vi "Custom.vi"(8 "error in (no error)":errorcluster, 11 "Transport Parameters in":T1 {"Serial Communication"."Baud Rate" items=["75"=75, "110"=110, "134"=134, "150"=150, "300"=300, "600"=600, "1200"=1200, "1800"=1800, "2400"=2400, "4800"=4800, "7200"=7200, "9600"=9600, "14400"=14400, "19200"=19200, "28800"=28800, "38400"=38400, "56000"=56000, "57600"=57600, "115200"=115200, "128000"=128000, "230400"=230400]}) -> (0 "error out":errorcluster, 3 "Transport Parameters out":T1 {"Serial Communication"."Baud Rate" items=["75"=75, "110"=110, "134"=134, "150"=150, "300"=300, "600"=600, "1200"=1200, "1800"=1800, "2400"=2400, "4800"=4800, "7200"=7200, "9600"=9600, "14400"=14400, "19200"=19200, "28800"=28800, "38400"=38400, "56000"=56000, "57600"=57600, "115200"=115200, "128000"=128000, "230400"=230400]})   [LabVIEW 2020]
uses:
  Controls/ConnectionParameters.ctl
  Controls/SupportedTransports.ctl
panel:
  out "spreadsheet string":string
  out "Message Out":string
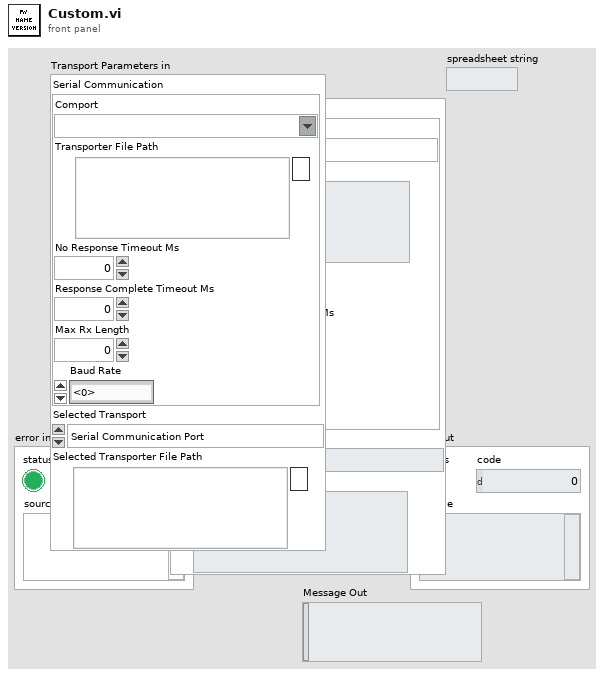
[diagram p1: front panel]
types:
  T1 = typedef "ConnectionParameters.ctl" = cluster{"Serial Communication":cluster{"Comport":refnum<visa-resource-name>, "Transporter File Path":path, "No Response Timeout Ms":u32, "Response Complete Timeout Ms":u32, "Max Rx Length":u32, "Baud Rate":u32}, "Selected Transport":T2, "Selected Transporter File Path":path}
  T2 = typedef "SupportedTransports.ctl" = enum16{"Serial Communication Port"}
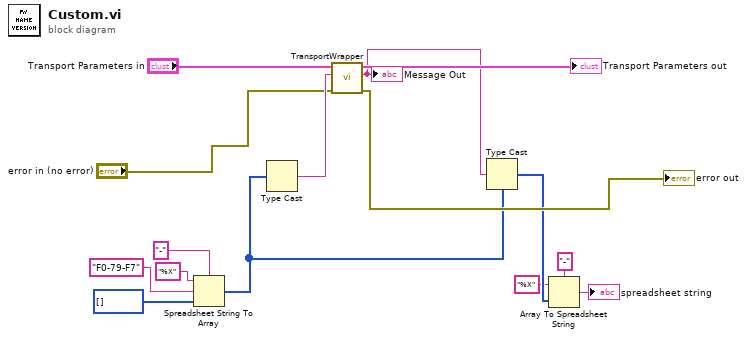
[diagram p0: block diagram]
diagram:
  n1 = Spreadsheet String To Array(delimiter (Tab)="-", format string="%X", spreadsheet string="F0-79-F7" ("Message In"), array type (2D Dbl)=u8[] []) -> (array=w5:u8[])
  n2 = Type Cast(x=w5) -> (*(type *) &x=w15:string)  [unwired: 1 in]
  n3 = call "TransportWrapper.vi"("error in"="error in (no error)", "Message In"=w15, "Transport Parameters In"="Transport Parameters in") -> ("error out"=→"error out":errorcluster, "Message Out"=w6:string, "Transport Parameters"=→"Transport Parameters out":T1)  [unwired: 6 in]
  "Message Out" <- w6
  n4 = Type Cast(type=w5, x=w6) -> (*(type *) &x=w4:u8[])
  n5 = Array To Spreadsheet String(delimiter (Tab)="-", array=w4, 3:"%X" ("format string")) -> (spreadsheet string=→"spreadsheet string":string)
